vi "get children.vi"(11 "communicator in":refnum<class "communicator.lvclass">) -> (3 "children":refnum<class "identifying queue.lvclass">[](array[class]))   [LabVIEW 2015, in "communicator.lvclass"]
uses:
  communicator.lvclass
  communicator queue/identifying queue.lvclass
  communicator.lvclass/communicator.ctl
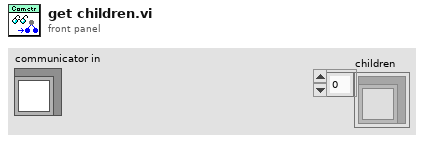
[diagram p1: front panel]
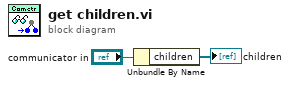
[diagram p0: block diagram]
diagram:
  n1 = Unbundle By Name("communicator in") -> ("children"=→"children":refnum<class "identifying queue.lvclass">[])
